vi "DataLog Bisection Search LE Point Times.vi"(0 "tag log directory":path, 1 "search timestamp":dbl format="%<%I:%M:%S %p\n%Y/%m/%d>T", 5 "min index (0)":i32, 7 "points":T1[](array[typedef]) {"value" format="%.3e"; "time" format="%<%H:%M:%S%2u\n%Y/%m/%d>T"}, 9 "max index (#points - 1)":i32=-1, 11 "error in (no error)":errorcluster) -> (4 "dup tag log directory":path, 6 "index":i32, 8 "dup points":T1[](array[typedef]) {"value" format="%.3e"; "time" format="%<%H:%M:%S%2u\n%Y/%m/%d>T"}, 10 "at max?":bool, 15 "error out":errorcluster)   [LabVIEW 2012]
doc: "Bisection searches an array of points. The timestamps of the points must be sorted in increasing order. The index into the chunk of the last point with timestamp <= the search timestamp is returned. This operation scales as log(N), where N is the number of points in the array. Some sanity checks are performed so as to ensure that the search always terminates."
uses:
  typedefs/clusters/t_DataLog Point.ctl
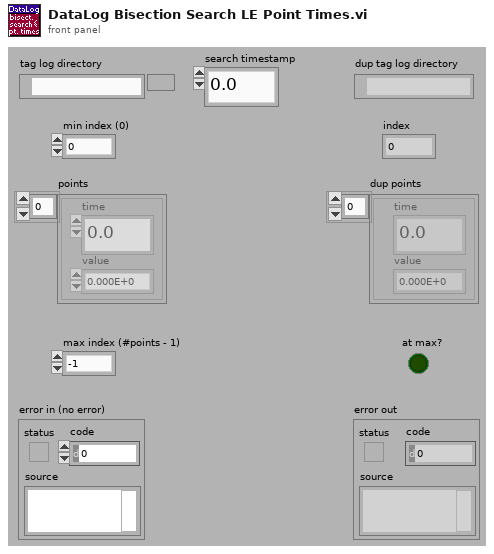
[diagram p1: front panel]
types:
  T1 = typedef "t_DataLog Point.ctl" = cluster{"time":dbl, "value":dbl}
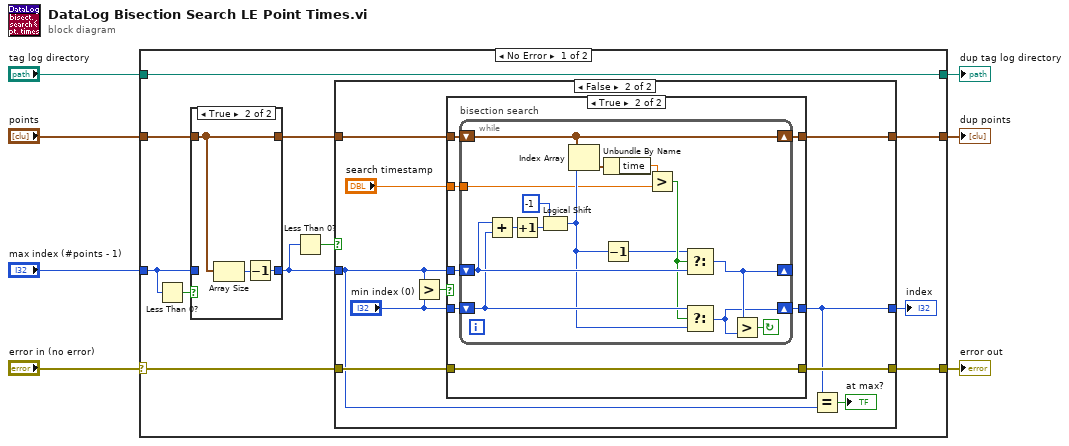
[diagram p0: block diagram]
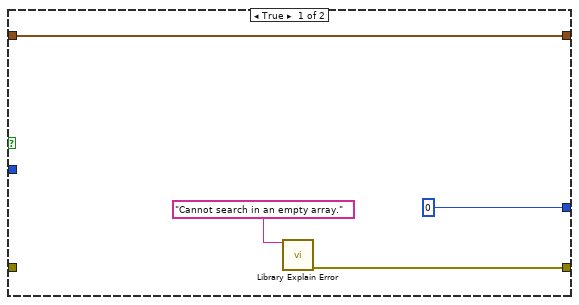
[diagram p3: hidden frame]
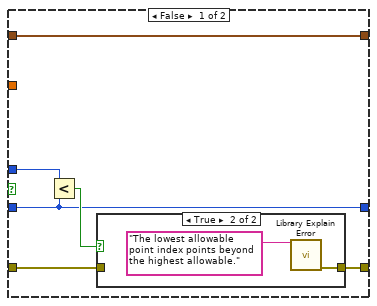
[diagram p4: hidden frame]
diagram:
  n1 = case shown="No Error" "error in (no error)" {
    selector: "error in (no error)" -> [w15 w71]
    tunnel: [w16 w71] -> w7
    tunnel: "tag log directory" -> [w18 w70]
    tunnel: [w18 w70] -> w4
    tunnel: "points" -> [w13 w69]
    tunnel: [w14 w69] -> w2
    tunnel: "max index (#points - 1)" -> [w10 _]
    frame No Error {
      n2 = Less Than 0?(x=w10) -> (x < 0?=w11:bool)
      n3 = case shown="True" w11 {
        tunnel: [w20 w21] -> w9
        tunnel: w13 -> [w19 w23]
        tunnel: [w19 w23] -> w12
        tunnel: w10 -> [w20 _]
        frame False {
        }
        frame True {
          n4 = Array Size(array=w23) -> (size(s)=w22:i32)
          n5 = Decrement(x=w22) -> (x-1=w21:i32)
        }
      }
      n6 = Less Than 0?(x=w9) -> (x < 0?=w8:bool)
      n7 = case shown="False" w8 {
        tunnel: [0 w28] -> w17
        tunnel: [w26 w33] -> w16
        tunnel: w15 -> [_ w34]
        tunnel: w12 -> [w24 w32]
        tunnel: [w24 w31] -> w14
        tunnel: w9 -> [_ w29]
        frame True {
          n8 = call "Library Explain Error.vi"("explanation prefix (none)"="Cannot search in an empty array." ("explanation")) -> ("explained error"=w26:errorcluster)  [unwired: 14 in]
        }
        frame False {
          n9 = Greater?(x=w29, y="min index (0)") -> (0:w35:bool)
          n10 = case shown="True" w35 {
            tunnel: "search timestamp" -> [_ w53]
            tunnel: w29 -> [w42 w48]
            tunnel: "min index (0)" -> [w38 w52]
            tunnel: w34 -> [w40 w51]
            tunnel: [w43 w51] -> w33
            tunnel: w32 -> [w39 w50]
            tunnel: [w39 w49] -> w31
            tunnel: [w38 w47] -> w28
            frame False {
              n11 = Less?(x=w42, y=w38) -> (x < y?=w41:bool)
              n12 = case shown="True" w41 {
                tunnel: [w44 w46] -> w43
                tunnel: w40 -> [w44 _]
                frame False {
                }
                frame True {
                  n13 = call "Library Explain Error.vi"("explanation prefix (none)"="The lowest allowable point index points beyond the highest allowable." ("explanation")) -> ("explained error"=w46:errorcluster)  [unwired: 14 in]
                }
              }
            }
            frame True {
              n14 = while "bisection search" {
                shift-right: [w60] -> w47
                shift-left: w52 -> [w67]
                shift-right: [w66] -> _
                shift-left: w48 -> [w68]
                tunnel: w53 -> [w57]
                shift-right: [w54] -> w49
                shift-left: w50 -> [w54]
                stop <- w65 continue-if-true
                n15 = Add(x=w68, y=w67) -> (x+y=w63:i32)
                n16 = Increment(x=w63) -> (x+1=w58:i32)
                n17 = Logical Shift(y=-1, x=w58) -> (x << y=w61:i32)
                n18 = Index Array(array=w54, index=w61) -> (element=w56:T1)
                n19 = Decrement(x=w61) -> (x-1=w59:i32)
                n20 = Unbundle By Name(w56) -> ("time"=w55:dbl)
                n21 = Greater?(x=w55, y=w57) -> (0:w64:bool)
                n22 = Select(t=w59, s=w64, f=w68) -> (s? t:f=w66:i32)
                n23 = Select(t=w67, s=w64, f=w61) -> (s? t:f=w60:i32)
                n24 = Greater?(x=w66, y=w60) -> (0:w65:bool)
              }
            }
          }
          n25 = Equal?(x=w28, y=w29) -> (x = y?=→"at max?":bool)
        }
      }
      "index" <- w17
    }
    frame Error {
    }
  }
  "error out" <- w7
  "dup tag log directory" <- w4
  "dup points" <- w2
